vi "encode point.vi"(10 "y":i16, 11 "x":i16) -> (1 "pixel send message":u8[](array[numeric]))   [LabVIEW 2009]
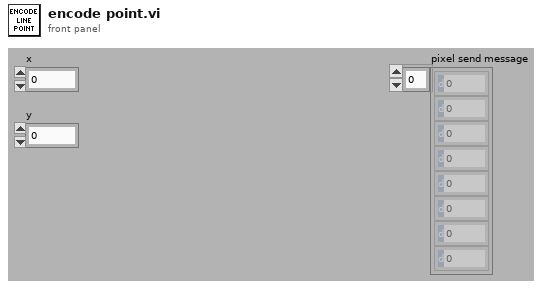
[diagram p1: front panel]
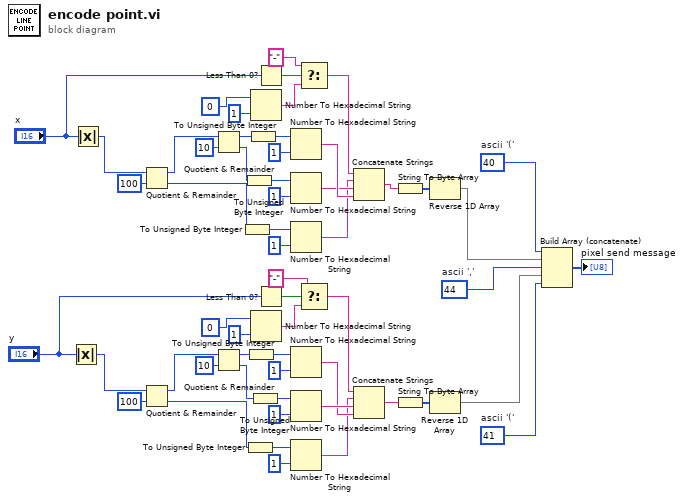
[diagram p0: block diagram]
diagram:
  w39 = u8 41  # ascii '('
  w56 = u8 40  # ascii '('
  w54 = u8 44  # ascii ','
  n1 = Absolute Value(x="y") -> (abs(x)=w22:i16)
  n2 = Absolute Value(x="x") -> (abs(x)=w24:i16)
  n3 = Quotient & Remainder(x=w24, y=i16 100) -> (x-y*floor(x/y)=w1:i16, floor(x/y)=w2:i16)
  n4 = Quotient & Remainder(x=w22, y=i16 100) -> (x-y*floor(x/y)=w3:i16, floor(x/y)=w4:i16)
  n5 = Quotient & Remainder(x=w1, y=i16 10) -> (x-y*floor(x/y)=w49:i16, floor(x/y)=w47:i16)
  n6 = Quotient & Remainder(x=w3, y=i16 10) -> (x-y*floor(x/y)=w30:i16, floor(x/y)=w32:i16)
  n7 = To Unsigned Byte Integer(number=w2) -> (unsigned 8bit integer=w7:u8)
  n8 = To Unsigned Byte Integer(number=w47) -> (unsigned 8bit integer=w6:u8)
  n9 = To Unsigned Byte Integer(number=w4) -> (unsigned 8bit integer=w8:u8)
  n10 = To Unsigned Byte Integer(number=w30) -> (unsigned 8bit integer=w10:u8)
  n11 = To Unsigned Byte Integer(number=w49) -> (unsigned 8bit integer=w5:u8)
  n12 = To Unsigned Byte Integer(number=w32) -> (unsigned 8bit integer=w9:u8)
  n13 = Number To Hexadecimal String(1:i16 1 ("width (-)"), 2:u8 0 ("f")) -> (0:w21:string)
  n14 = Number To Hexadecimal String(1:i16 1 ("width (-)"), 2:u8 0 ("f")) -> (0:w16:string)
  n15 = Less Than 0?(x="x") -> (x < 0?=w44:bool)
  n16 = Less Than 0?(x="y") -> (x < 0?=w14:bool)
  n17 = Number To Hexadecimal String(1:i16 1 ("width (-)"), 2:w5) -> (0:w38:string)
  n18 = Number To Hexadecimal String(1:i16 1 ("width (-)"), 2:w6) -> (0:w37:string)
  n19 = Number To Hexadecimal String(1:i16 1 ("width (-)"), 2:w7) -> (0:w26:string)
  n20 = Number To Hexadecimal String(1:i16 1 ("width (-)"), 2:w10) -> (0:w35:string)
  n21 = Number To Hexadecimal String(1:i16 1 ("width (-)"), 2:w9) -> (0:w36:string)
  n22 = Number To Hexadecimal String(1:i16 1 ("width (-)"), 2:w8) -> (0:w25:string)
  n23 = Select(t="-", s=w44, f=w21) -> (s? t:f=w11:string)
  n24 = Select(t="-", s=w14, f=w16) -> (s? t:f=w12:string)
  n25 = Concatenate Strings(w11, w26, w37, w38) -> (w45:string)
  n26 = Concatenate Strings(w12, w25, w36, w35) -> (w27:string)
  n27 = String To Byte Array(string=w45) -> (unsigned byte array=w55:u8[])
  n28 = String To Byte Array(string=w27) -> (unsigned byte array=w41:u8[])
  n29 = Reverse 1D Array(array=w55) -> (reversed array=w53:u8[])
  n30 = Reverse 1D Array(array=w41) -> (reversed array=w40:u8[])
  n31 = Build Array (concatenate)(w56, w53, w54, w40, w39) -> (→"pixel send message":u8[])
